vi "InitializeSerialPort.vi"(2 "error in (no error)":errorcluster, 3 "Serial Port to Use":refnum<visa-resource-name>="COM8") -> (0 "error out":errorcluster, 1 "Configured Serial Port Identifier":refnum<visa-resource-name>)   [LabVIEW 2012]
uses:
  <vilib>/Instr/_visa.llb/VISA Configure Serial Port (Instr).vi
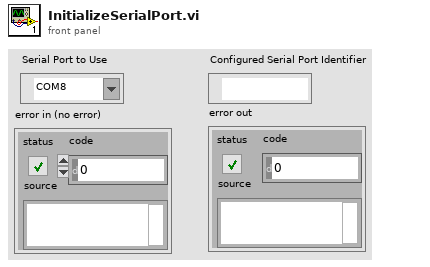
[diagram p1: front panel]
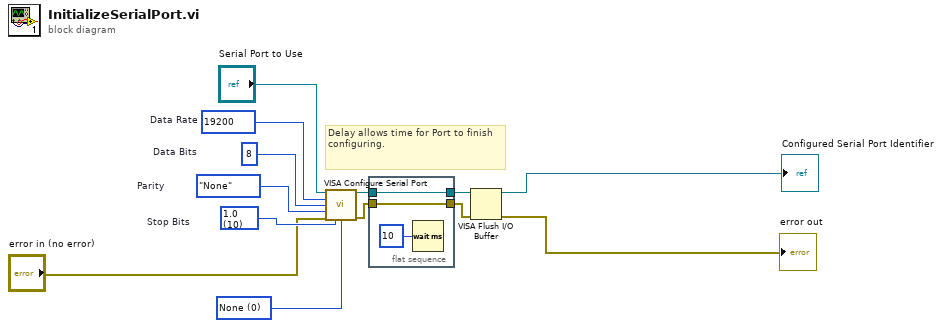
[diagram p0: block diagram]
diagram:
  w8 = u16 0 items=["None", "XON/XOFF", "RTS/CTS", "XON/XOFF & RTS/CTS", "DTR/DSR", "XON/XOFF & DTR/DSR"] ("flow control (0:none)")
  w10 = u16 10 items=["1.0"=10, "1.5"=15, "2.0"=20]  # Stop Bits
  w11 = enum16{"None", "Odd", "Even", "Mark", "Space"}."None"  # Parity
  w12 = u16 8  # Data Bits
  w13 = u32 19200  # Data Rate
  # "Delay allows time for Port to finish configuring."
  n1 = call-poly "VISA Configure Serial Port"("VISA resource name"="Serial Port to Use", "baud rate (9600)"=w13, "data bits (8)"=w12, "parity (0:none)"=w11, "error in (no error)"="error in (no error)", "stop bits (10: 1 bit)"=w10, "flow control (0:none)"=w8) -> ("VISA resource name out"=w6:refnum<visa-resource-name>, "error out"=w5:errorcluster)  [unwired: 7 in]
  n2 = flat-sequence {
    tunnel: w6 -> [w14]
    tunnel: w5 -> [w15]
    tunnel: [w15] -> w3
    tunnel: [w14] -> w4
    frame #0 {
      n3 = Wait (ms)(milliseconds to wait=u32 10) -> ()  [unwired: 1 out]
    }
  }
  n4 = VISA Flush I/O Buffer(VISA resource name=w4, error in (no error)=w3) -> (VISA resource name out=→"Configured Serial Port Identifier":refnum<visa-resource-name>, error out=→"error out":errorcluster)  [unwired: 1 in]
